vi "INIScoreFile Get Strings.vi"(8 "error in (no error)":errorcluster, 11 "INIScoreFile in":refnum<class "INIScoreFile.lvclass">) -> (0 "error out":errorcluster, 2 "Lines":string[](array[string]), 3 "INIScoreFile out":refnum<class "INIScoreFile.lvclass">)   [LabVIEW 2020, in "INIScoreFile.lvclass"]
uses:
  INIScoreFile.lvclass
  INIScoreFile.lvclass/INIScoreFile.ctl
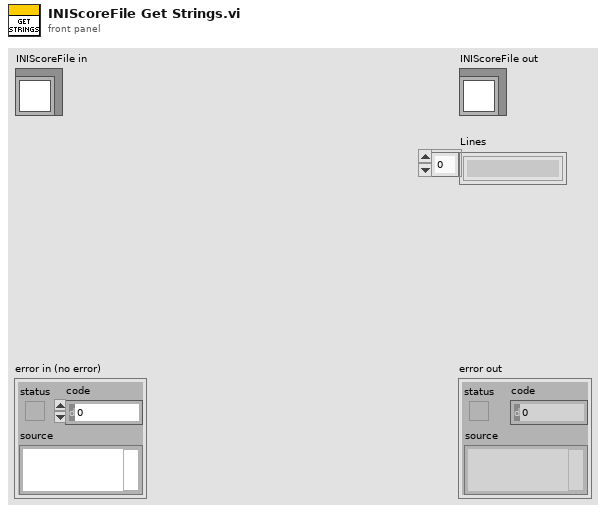
[diagram p1: front panel]
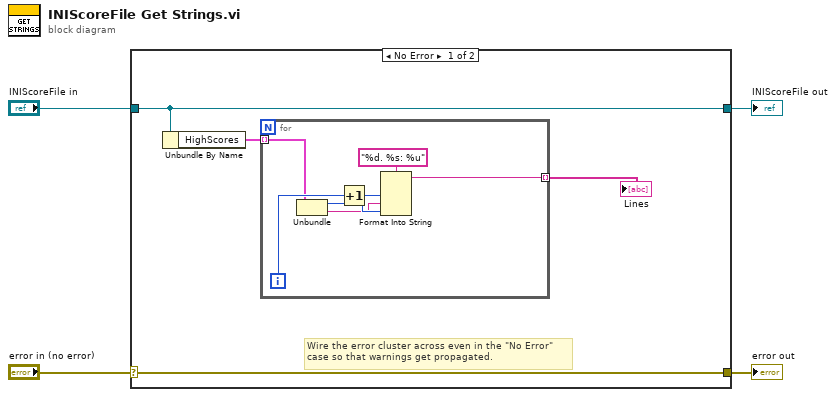
[diagram p0: block diagram]
diagram:
  n1 = case shown="No Error" "error in (no error)" {
    selector: "error in (no error)" -> [w8 w17]
    tunnel: [w8 w17] -> w3
    tunnel: [w7 w16] -> w1
    tunnel: "INIScoreFile in" -> [w7 w16]
    frame No Error {
      # "Wire the error cluster across even in the \"No Error\"\ncase so that warnings get propagated."
      n2 = Unbundle By Name(w7) -> ("HighScores"=w6:cluster{"Score":u32, "Name":string}[])
      n3 = for {
        tunnel: w6 -> [w13] mode=indexing
        tunnel: [w10] -> w5 mode=indexing
        i -> [w14]
        n4 = Unbundle(w13) -> ("Score"=w12:u32, "Name"=w11:string)
        n5 = Increment(x=w14) -> (x+1=w9:i32)
        n6 = Format Into String(format string="%d. %s: %u", w9, w11, w12) -> (resulting string=w10:string)  [unwired: 2 in, 1 out]
      }
      "Lines" <- w5
    }
    frame Error {
    }
  }
  "error out" <- w3
  "INIScoreFile out" <- w1
